vi "Initialize NI-DAQ continuous recorder.vi"(8 "error in (no error)":errorcluster, 11 "Parameters":T1={"physical channels"="Dev1/ai0:7", "input terminal configuration"=10106, "Range"=10.0, "Sample rate"=1000000.0, "samples per channel"=220000, "Trigger source"="/Dev1/PFI0", "pretrigger samples per channel"=20000, "task"="", "Sample mode"=10178, "Retriggerable"=FALSE, "File Path"=path ""} {"Sample mode" items=["Finite Samples"=10178, "Continuous Samples"=10123, "Hardware Timed Single Point"=12522]; "Sample rate" format="%.2p"; "input terminal configuration" items=["default"=-1, "RSE"=10083, "NRSE"=10078, "Differential"=10106, "Pseudodifferential"=12529]}) -> (0 "error out":errorcluster, 3 "Parameters out":T1={"physical channels"="Dev1/ai0:7", "input terminal configuration"=10106, "Range"=10.0, "Sample rate"=1000000.0, "samples per channel"=220000, "Trigger source"="/Dev1/PFI0", "pretrigger samples per channel"=20000, "task"="", "Sample mode"=10178, "Retriggerable"=FALSE, "File Path"=path ""} {"Sample mode" items=["Finite Samples"=10178, "Continuous Samples"=10123, "Hardware Timed Single Point"=12522]; "Sample rate" format="%.2p"; "input terminal configuration" items=["default"=-1, "RSE"=10083, "NRSE"=10078, "Differential"=10106, "Pseudodifferential"=12529]})   [LabVIEW 2015]
uses:
  NI-DAQ digitizer parameters.ctl
  <vilib>/DAQmx/create/channels.llb/DAQmx Create Channel (AI-Voltage-Basic).vi
  <vilib>/DAQmx/configure/timing.llb/DAQmx Timing (Sample Clock).vi
  <vilib>/DAQmx/configure/trigger.llb/DAQmx Reference Trigger (Digital Edge).vi
  <vilib>/DAQmx/configure/task.llb/DAQmx Configure Logging (TDMS).vi
  <resource>/objmgr/daqmx.rc
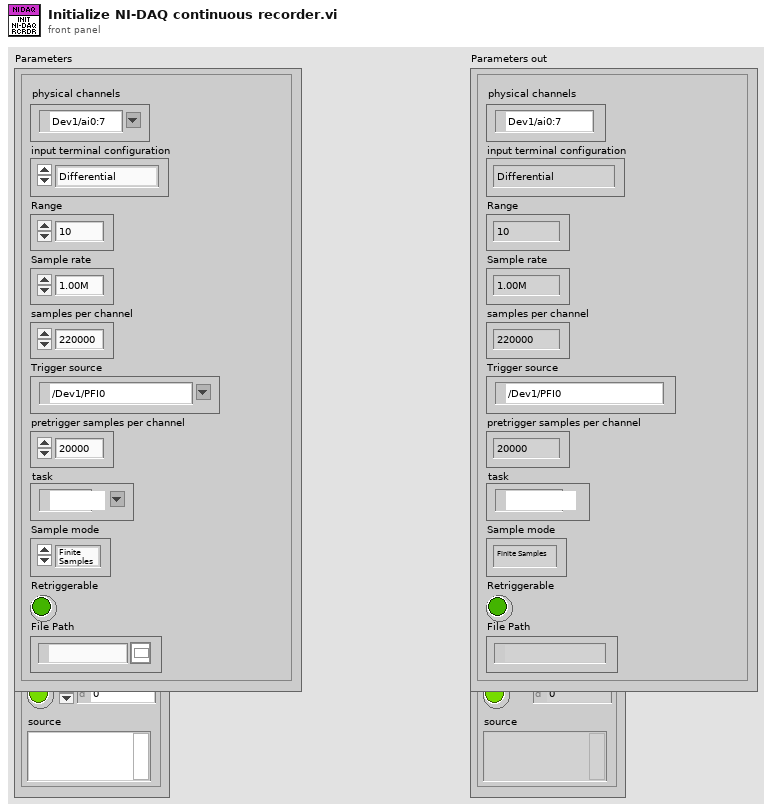
[diagram p1: front panel]
types:
  T1 = typedef "NI-DAQ digitizer parameters.ctl" = cluster{"physical channels":tag, "input terminal configuration":i32, "Range":dbl, "Sample rate":dbl, "samples per channel":i32, "Trigger source":tag, "pretrigger samples per channel":u32, "task":refnum<k21>, "Sample mode":i32, "Retriggerable":bool, "File Path":path}
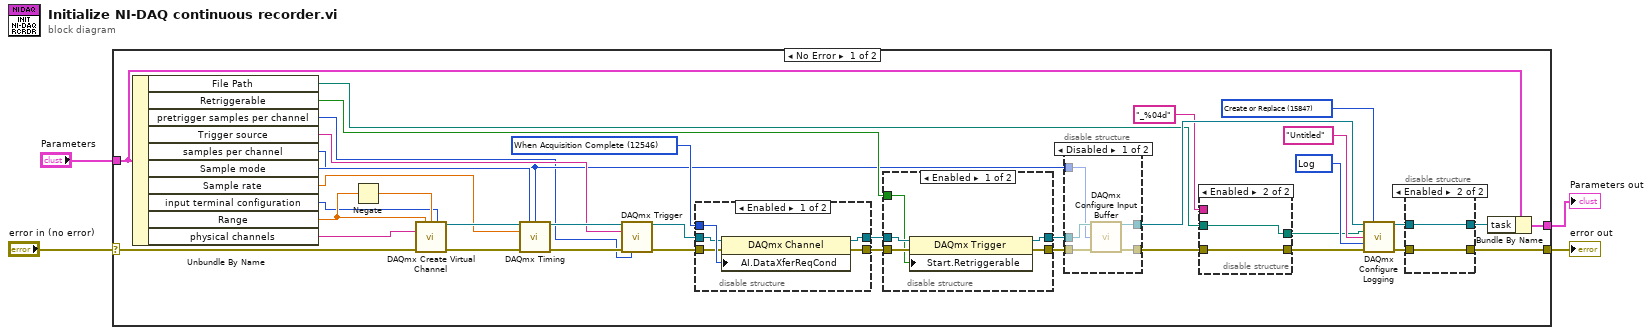
[diagram p0: block diagram]
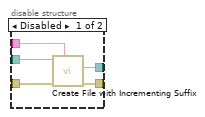
[diagram p2: hidden frame]
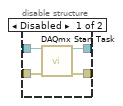
[diagram p3: hidden frame]
diagram:
  n1 = case shown="No Error" "error in (no error)" {
    selector: "error in (no error)" -> [w21 w77]
    tunnel: [w19 w77] -> w1
    tunnel: [w29 w76] -> w2
    tunnel: "Parameters" -> [w22 w76]
    frame No Error {
      w12 = 15847 items=["Open"=10437, "Open or Create"=15846, "Create or Replace"=15847, "Create"=15848] ("Logging.TDMS.Operation")
      w10 = 15844 items=["Off"=10231, "Log"=15844, "Log and Read"=15842] ("Logging.Mode")
      w27 = 12546 items=["Onboard Memory More than Half Full"=10237, "Onboard Memory Not Empty"=10241, "Onboard Memory Custom Threshold"=12577, "When Acquisition Complete"=12546] ("AI.DataXferReqCond")
      n2 = Unbundle By Name(w22) -> ("File Path"=w7:path, "Retriggerable"=w30:bool, "pretrigger samples per channel"=w15:u32, "Trigger source"=w31:tag, "samples per channel"=w16:i32, "Sample mode"=w32:i32, "Sample rate"=w33:dbl, "input terminal configuration"=w34:i32, "Range"=w35:dbl, "physical channels"=w36:tag)
      n3 = Negate(x=w35) -> (-x=w41:dbl)
      n4 = call-poly <vilib>:"DAQmx Create Virtual Channel.vi"("maximum value"=w35, "minimum value"=w41, "input terminal configuration"=w34, "physical channels"=w36, "error in"=w21) -> ("task out"=w40:refnum<k21>, "error out"=w39:errorcluster)  [unwired: 4 in, 5 out]
      n5 = call-poly <vilib>:"DAQmx Timing.vi"("task/channels in"=w40, "sample mode"=w32, "samples per channel"=w16, "rate"=w33, "error in"=w39) -> ("task out"=w38:refnum<k21>, "error out"=w37:errorcluster)  [unwired: 9 in]
      n6 = call-poly <vilib>:"DAQmx Trigger.vi"("task/channels in"=w38, "source"=w31, "error in"=w37, "pretrigger samples per channel"=w15) -> ("task out"=w26:refnum<k21>, "error out"=w23:errorcluster)  [unwired: 1 in, 9 out]
      n7 = disable-structure shown="Enabled" {
        disable-tunnel: w27 -> [w66 _]
        disable-tunnel: w26 -> [w65 w67]
        disable-tunnel: [w64 w67] -> w25
        disable-tunnel: [w63 w68] -> w24
        disable-tunnel: w23 -> [w62 w68]
        frame Enabled {
          n8 = property class="DAQmx Channel"(reference=w65, error in=w62, "AI.DataXferReqCond"=w66) -> (reference out=w64:refnum<k21>, error out=w63:errorcluster)
        }
        frame Disabled {
        }
      }
      n9 = disable-structure shown="Enabled" {
        disable-tunnel: w24 -> [w73 w75]
        disable-tunnel: w25 -> [w72 w74]
        disable-tunnel: [w71 w75] -> w17
        disable-tunnel: w30 -> [w70 _]
        disable-tunnel: [w69 w74] -> w28
        frame Enabled {
          n10 = property class="DAQmx Trigger"(reference=w72, error in=w73, "Start.Retriggerable"=w70) -> (reference out=w69:refnum<k21>, error out=w71:errorcluster)
        }
        frame Disabled {
        }
      }
      n11 = disable-structure shown="Disabled" {
        disable-tunnel: w28 -> [w59 w60]
        disable-tunnel: [w58 w60] -> w18
        disable-tunnel: w16 -> [w57 _]
        disable-tunnel: [w56 w61] -> w8
        disable-tunnel: w17 -> [w55 w61]
        frame Disabled {
          n12 = call <vilib>:"DAQmx Configure Input Buffer.vi"("task/channels in"=w59, "buffer size (in samples per channel)"=w57, "error in"=w55) -> ("task out"=w58:refnum<k21>, "error out"=w56:errorcluster)  [unwired: 11 in]
        }
        frame Enabled {
        }
      }
      n13 = disable-structure shown="Enabled" {
        disable-tunnel: [w46 w47] -> w9
        disable-tunnel: w8 -> [w45 w47]
        disable-tunnel: w7 -> [w44 w48]
        disable-tunnel: "_%04d" ("format string (\" (%d)\")") -> [w43 _]
        disable-tunnel: [w42 w48] -> w5
        frame Disabled {
          n14 = call <vilib>:"Create File with Incrementing Suffix.vi"("format string (\" (%d)\")"=w43, "error in (no error)"=w45, "file path"=w44) -> ("error out"=w46:errorcluster, "actual path"=w42:path)  [unwired: 6 in, 1 out]
        }
        frame Enabled {
        }
      }
      n15 = call-poly <vilib>:"DAQmx Configure Logging.vi"("task/channels in"=w18, "operation"=w12, "file path"=w5, "group name"="Untitled" ("Logging.TDMS.GroupName"), "logging mode"=w10, "error in"=w9) -> ("task out"=w14:refnum<k21>, "error out"=w13:errorcluster)  [unwired: 8 in]
      n16 = disable-structure shown="Enabled" {
        disable-tunnel: [w52 w53] -> w20
        disable-tunnel: [w51 w54] -> w19
        disable-tunnel: w14 -> [w50 w53]
        disable-tunnel: w13 -> [w49 w54]
        frame Disabled {
          n17 = call <vilib>:"DAQmx Start Task.vi"("task/channels in"=w50, "error in"=w49) -> ("task out"=w52:refnum<k21>, "error out"=w51:errorcluster)  [unwired: 12 in]
        }
        frame Enabled {
        }
      }
      n18 = Bundle By Name(cluster=w22, "task"=w20) -> (w29:T1)
    }
    frame Error {
    }
  }
  "error out" <- w1
  "Parameters out" <- w2
